vi "Teleop.vi"(10 "Match Info":T1={"Autonomous Elapsed Seconds"=0.0, "TeleOp Elapsed Seconds"=0.0, "Disabled Elapsed Seconds"=0.0, "Visited Autonomous"=FALSE, "Visited TeleOp"=FALSE, "Visited Disabled"=FALSE, "Autonomous Settings"={"Autonomous Style"=enum."Independent", "VI Refnum"=refnum}}, 11 "Call Context":T2) -> ()   [LabVIEW 2019]
doc: "This VI is called for each TeleOp packet received from the DS where the robot is not disabled. It is often used to read from the joysticks and update I/O or to update setpoints for timed control loops. It should complete and return within 20 milliseconds or it may miss DS packets."
uses:
  <vilib>/Rock Robotics/WPI/DriverStation/WPI_DriverStationDerivedRobotMode.ctl
  <vilib>/Rock Robotics/WPI/DriverStation/WPI_DriverStationMatch Info.ctl
  <vilib>/Rock Robotics/WPI/Utilities/WPI_GetSetVariantRefNum.vi
  <vilib>/Rock Robotics/Network Tables/NT Write Boolean Array.vi
  <vilib>/Rock Robotics/Network Tables/NT Write Numeric Array.vi
  <vilib>/Rock Robotics/Network Tables/NT Read Boolean.vi
  <vilib>/Rock Robotics/Network Tables/NT Read Number.vi
  <vilib>/Rock Robotics/WPI/Ultrasonic/WPI_UltrasonicRangeUnits.ctl
  <vilib>/Rock Robotics/WPI/Ultrasonic/WPI_SonarSRF04DigitalGetRange.vi
  <vilib>/Rock Robotics/WPI/Ultrasonic/WPI_SonarSRF04DigitalRefNum Registry Get.vi
panel:
  out "Numeric 3":dbl
  out "Numeric 2":dbl
  out "RSL":bool
  out "Angle":dbl(knob) scale=0.0..360.0
  out "Gyro":i32
  out "Ultrasonic":dbl
  out "Sample Slider 0":dbl(slide) scale=0.0..5.0
  out "Sample Boolean 1":bool
  out "Sample Boolean 0":bool
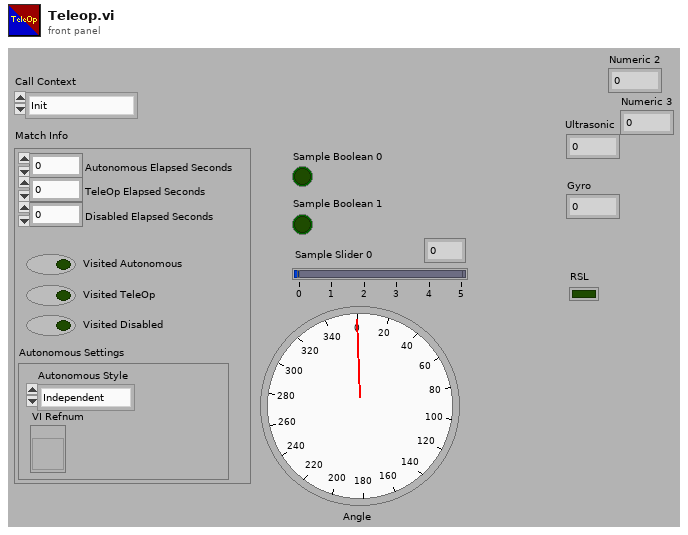
[diagram p1: front panel]
types:
  T1 = typedef "WPI_DriverStationMatch Info.ctl" = cluster{"Autonomous Elapsed Seconds":dbl, "TeleOp Elapsed Seconds":dbl, "Disabled Elapsed Seconds":dbl, "Visited Autonomous":bool, "Visited TeleOp":bool, "Visited Disabled":bool, "Autonomous Settings":cluster{"Autonomous Style":enum16{"Iterative", "Independent"}, "VI Refnum":refnum<vi>}}
  T2 = typedef "WPI_DriverStationDerivedRobotMode.ctl" = enum16{"Init", "Execute", "Stop"}
  T3 = typedef "WPI_RobotDriveDevRef.ctl" = cluster{"DevStatus":errorcluster, "Motors[]":T4[], "Square Inputs":bool, "Max Output":dbl}
  T4 = typedef "WPI_MotorControlDeviceRef.ctl" = cluster{"DeviceStatus":errorcluster, "Type":T5, "PWM":cluster{"PWM Channel":T6, "DeadBand":T7}, "CAN":cluster{"Device Number":u8, "SetOutput VI Ref":variant, "GetOutput VI Ref":variant, "Enable VI Ref":variant, "Disable VI Ref":variant, "Data":variant}, "Invert":bool, "DIO PWM":cluster{"PWM \"Enable\" Channel":T6, "DIOChannel":T8, "PWM Rate":dbl}}
  T5 = typedef "WPI_MotorControlType.ctl" = enum16{"PWM", "CAN", "DIO PWM"}
  T6 = typedef "FPGA_DIOPWMChannel.ctl" = enum8{"PWM 0", "PWM 1", "PWM 2", "PWM 3", "PWM 4", "PWM 5", "PWM 6", "PWM 7", "PWM 8", "PWM 9", "PWM MXP 0", "PWM MXP 1", "PWM MXP 2", "PWM MXP 3", "PWM MXP 4", "PWM MXP 5", "PWM MXP 6", "PWM MXP 7", "PWM MXP 8", "PWM MXP 9", "Invalid"}
  T7 = typedef "WPI_PWMDeadband.ctl" = cluster{"Name":string, "maxPositivePwm":i32, "minPositivePwm":i32, "centerPwm":i32, "maxNegativePwm":i32, "minNegativePwm":i32, "angularRange":u16}
  T8 = typedef "FPGA_DIOChannel.ctl" = enum8{"DIO 0", "DIO 1", "DIO 2", "DIO 3", "DIO 4", "DIO 5", "DIO 6", "DIO 7", "DIO 8", "DIO 9", "DIO MXP 0", "DIO MXP 1", "DIO MXP 2", "DIO MXP 3", "DIO MXP 4", "DIO MXP 5", "DIO MXP 6", "DIO MXP 7", "DIO MXP 8", "DIO MXP 9", "DIO MXP 10", "DIO MXP 11", "DIO MXP 12", "DIO MXP 13", "DIO MXP 14", "DIO MXP 15", "SPI Port CS1", "SPI Port CS2", "SPI Port CS3", "SPI Port MISO", "SPI Port MOSI", "Invalid"}
  T9 = typedef "WPI_JoystickDevRef.ctl" = cluster{"Device":T10}
  T10 = typedef "WPI_JoystickDeviceEnum.ctl" = enum16{"USB 0", "USB 1", "USB 2", "USB 3", "USB 4", "USB 5"}
  T11 = typedef "WPI_DigitalOutputDevRef.ctl" = cluster{"DIO Channel":T8, "DevStatus":errorcluster}
  T12 = typedef "WPI_UltrasonicRangeUnits.ctl" = enum16{"inches", "mm"}
  T13 = typedef "WPI_I2CDevRef.ctl" = cluster{"DevStatus":errorcluster, "Device Address":u8, "Handle":i32, "I2C Bus":T14}
  T14 = typedef "i2c_bus.ctl" = enum16{"I2C On-Board", "I2C MXP", "Invalid"}
  T15 = typedef "WPI_UltrasonicDeviceRef.ctl" = cluster{"DevStatus":errorcluster, "Ping Channel":T8, "Echo Channel":T8, "CntIndex":T16}
  T16 = typedef "FPGA_CounterCtrSystemIndex.ctl" = enum8{"Ctr 0", "Ctr 1", "Ctr 2", "Ctr 3", "Ctr 4", "Ctr 5", "Ctr 6", "Ctr 7", "Invalid"}
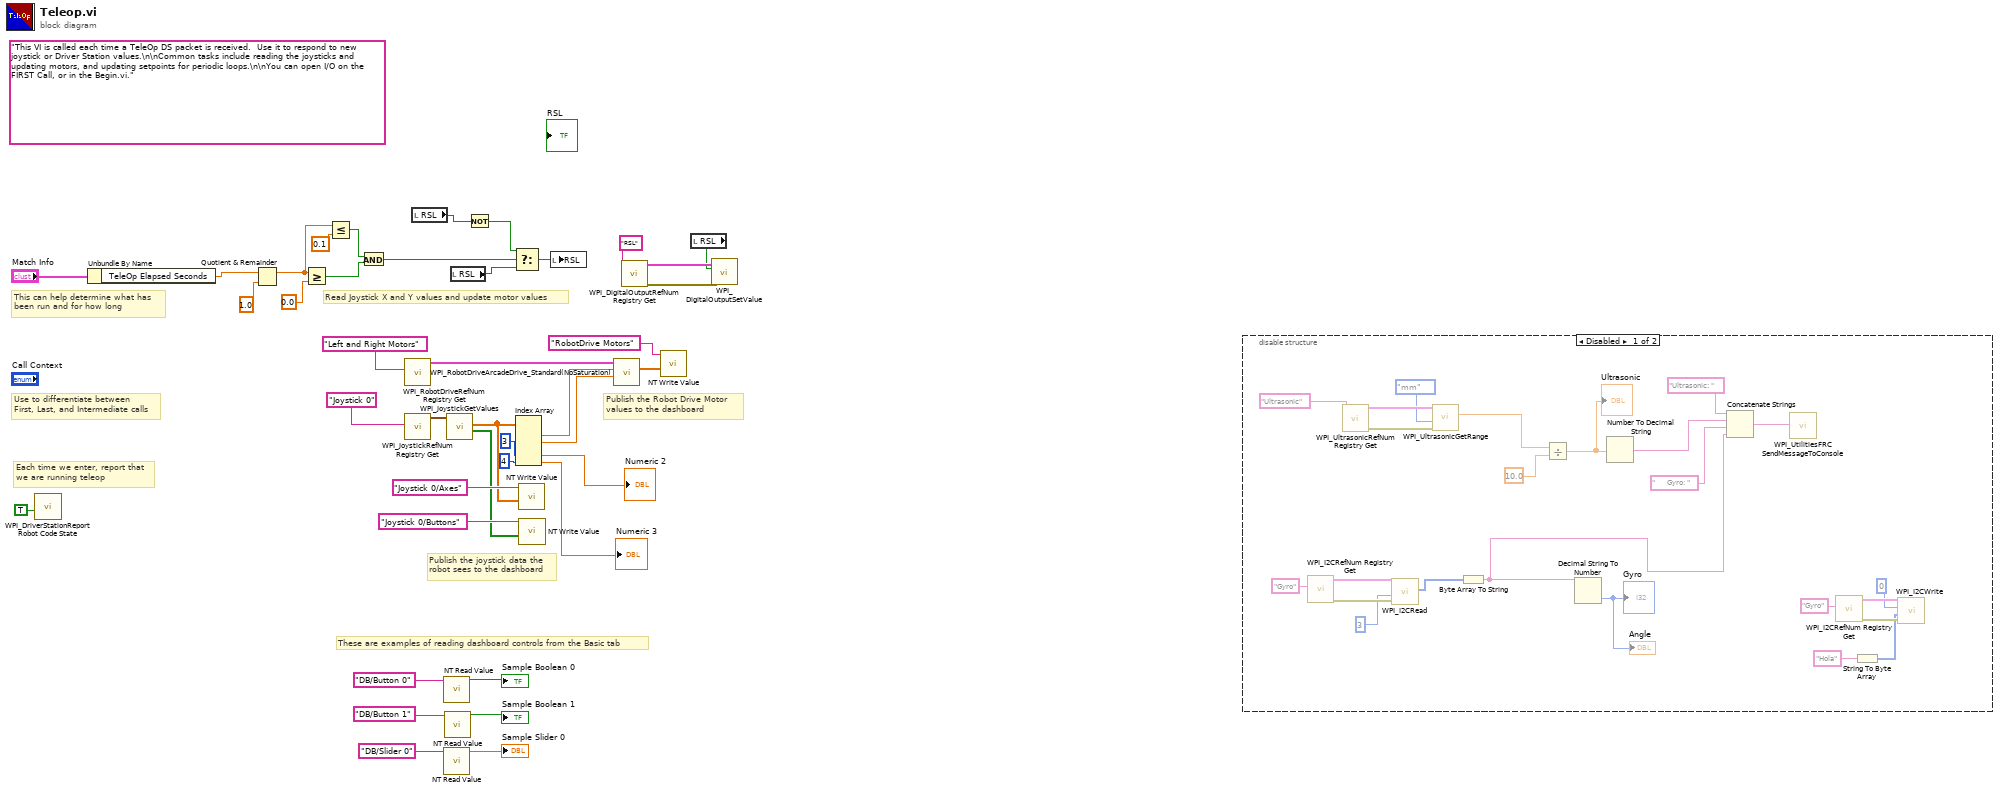
[diagram p0: block diagram]
diagram:
  (unwired) "This VI is called each time a TeleOp DS packet is received.  Use it to respond to new joystick or Driver Station values.\n\nCommon tasks include reading the joysticks and updating motors, and updating setpoints for periodic loops.\n\nYou can open I/O on the FIRST Call, or in the Begin.vi."
  # "These are examples of reading dashboard controls from the Basic tab"
  # "Publish the Robot Drive Motor\nvalues to the dashboard"
  # "Publish the joystick data the\nrobot sees to the dashboard"
  # "Each time we enter, report that\nwe are running teleop"
  # "Use to differentiate between\nFirst, Last, and Intermediate calls"
  # "This can help determine what has\nbeen run and for how long"
  # "Read Joystick X and Y values and update motor values"
  n1 = call <vilib>:"WPI_DriverStationReport Robot Code State.vi"("TeleOp"=TRUE ("Autonomous")) -> ()  [unwired: 10 in, 1 out]
  n2 = Unbundle By Name("Match Info") -> ("TeleOp Elapsed Seconds"=w20:dbl)
  n3 = Quotient & Remainder(x=w20, y=1.0) -> (x-y*floor(x/y)=w9:dbl)  [unwired: 1 out]
  n4 = Greater Or Equal?(x=w9, y=0.0) -> (x >= y?=w5:bool)
  n5 = Less Or Equal?(x=w9, y=0.1) -> (x <= y?=w6:bool)
  n6 = And(x=w6, y=w5) -> (x .and. y?=w7:bool)
  n7 = call <vilib>:"WPI_RobotDriveRefNum Registry Get.vi"("refnum name"="Left and Right Motors") -> ("RobotDriveDevRef"=w38:T3)  [unwired: 1 in, 9 out]
  n8 = call <vilib>:"WPI_JoystickRefNum Registry Get.vi"("refnum name"="Joystick 0") -> ("JoystickDevRef"=w35:T9)  [unwired: 1 in, 9 out]
  n9 = local read "RSL"() -> (w14:bool)
  n10 = call-poly <vilib>:"NT Read Value.vi"("Name"="DB/Button 0" ("refnum name")) -> ("Boolean"=→"Sample Boolean 0":bool)  [unwired: 9 in, 1 out]
  n11 = call-poly <vilib>:"NT Read Value.vi"("Name"="DB/Slider 0" ("refnum name")) -> ("Numeric"=→"Sample Slider 0":dbl)  [unwired: 9 in, 1 out]
  n12 = call-poly <vilib>:"NT Read Value.vi"("Name"="DB/Button 1" ("refnum name")) -> ("Boolean"=→"Sample Boolean 1":bool)  [unwired: 9 in, 1 out]
  n13 = call <vilib>:"WPI_JoystickGetValues.vi"("JoystickDevRef"=w35) -> ("Buttons"=w21:bool[], "Axes"=w30:dbl[])  [unwired: 6 in, 3 out]
  n14 = local read "RSL"() -> (w15:bool)
  n15 = Not(x=w14) -> (.not. x?=w13:bool)
  n16 = Select(t=w13, s=w7, f=w15) -> (s? t:f=w12:bool)
  n17 = Index Array(array=w30, index #4=3 ("index"), index #5=4 ("index")) -> (element #1=w37:dbl, element #2=w33:dbl, element #4=→"Numeric 2":dbl, element #5=→"Numeric 3":dbl)  [unwired: 3 in, 1 out]
  n18 = call-poly <vilib>:"NT Write Value.vi"("Numeric Array"=w30, "Name"="Joystick 0/Axes") -> ()  [unwired: 9 in, 1 out]
  n19 = call-poly <vilib>:"NT Write Value.vi"("Boolean Array"=w21, "Name"="Joystick 0/Buttons") -> ()  [unwired: 9 in, 1 out]
  n20 = local write "RSL"(w12) -> ()
  n21 = call <vilib>:"WPI_RobotDriveArcadeDrive_Standard(NoSaturation).vi"("Y axis value"=w33, "X axis value"=w37, "RobotDriveDevRef"=w38) -> ("Motor Values"=w23:dbl[])  [unwired: 1 in, 7 out]
  n22 = call <vilib>:"WPI_DigitalOutputRefNum Registry Get.vi"("refnum name"="RSL") -> ("error out"=w17:errorcluster, "DigitalOutputDevRef"=w18:T11)  [unwired: 9 in]
  n23 = call-poly <vilib>:"NT Write Value.vi"("Numeric Array"=w23, "Name"="RobotDrive Motors") -> ()  [unwired: 9 in, 1 out]
  n24 = local read "RSL"() -> (w16:bool)
  n25 = call <vilib>:"WPI_DigitalOutputSetValue.vi"("error in (no error)"=w17, "Value"=w16, "DigitalOutputDevRef"=w18) -> ()  [unwired: 7 in, 2 out]
  n26 = disable-structure shown="Disabled" {
    frame Disabled {
      n27 = call <vilib>:"WPI_I2CRefNum Registry Get.vi"("refnum name"="Gyro") -> ("error out"=w62:errorcluster, "I2CDevRef"=w63:T13)  [unwired: 9 in]
      n28 = call-poly <vilib>:"WPI_UltrasonicRefNum Registry Get.vi"("refnum name"="Ultrasonic") -> ("error out"=w56:errorcluster, "SonarSRF04DevRef"=w57:T15)  [unwired: 9 in]
      n29 = call <vilib>:"WPI_I2CRead.vi"("error in (no error)"=w62, "I2CBytesToRead"=u8 3, "I2CDevRef"=w63) -> ("Data Out"=w59:u8[])  [unwired: 6 in, 2 out]
      n30 = call-poly <vilib>:"WPI_UltrasonicGetRange.vi"("error in (no error)"=w56, "Range Units"=WPI_UltrasonicRangeUnits."mm", "SonarSRF04DevRef"=w57) -> ("Distance"=w53:dbl)  [unwired: 6 in, 2 out]
      n31 = Byte Array To String(unsigned byte array=w59) -> (string=w64:string)
      n32 = Divide(x=w53, y=10.0) -> (x/y=w47:dbl)
      "Ultrasonic" <- w47
      n33 = Decimal String To Number(string=w64) -> (number=→"Gyro" →"Angle":i32)  [unwired: 2 in, 1 out]
      n34 = Number To Decimal String(number=w47) -> (decimal integer string=w50:string)  [unwired: 1 in]
      n35 = Concatenate Strings("Ultrasonic: " ("string"), w50, "      Gyro: " ("string"), w64) -> (w48:string)
      n36 = call <vilib>:"WPI_UtilitiesFRC SendMessageToConsole.vi"("Message"=w48) -> ()  [unwired: 14 in, 1 out]
      n37 = call <vilib>:"WPI_I2CRefNum Registry Get.vi"("refnum name"="Gyro") -> ("error out"=w44:errorcluster, "I2CDevRef"=w45:T13)  [unwired: 9 in]
      n38 = String To Byte Array(string="Hola") -> (unsigned byte array=w43:u8[])
      n39 = call <vilib>:"WPI_I2CWrite.vi"("error in (no error)"=w44, "I2CDataToSend"=w43, "I2CRegister"=u8 0, "I2CDevRef"=w45) -> ()  [unwired: 6 in, 2 out]
    }
    frame Enabled {
    }
  }
